vi "testFlushQueueTcpClient.vi"(8 "error in (no error)":errorcluster) -> (0 "error out":errorcluster)   [LabVIEW 2018]
doc: "Test the flushQueueTcpClient.vi."
uses:
  src/TcpServerBase/TcpServerBase.lvclass
  src/TcpServerBase/TcpServerBase.lvclass/TcpServerBase.ctl
  <vilib>/addons/_JKI Toolkits/Caraya/classes/Assert/Assert True.vi
  <vilib>/addons/_JKI Toolkits/Caraya/classes/Test/Test.lvclass
  <vilib>/addons/_JKI Toolkits/Caraya/classes/Assert/Assert.lvclass
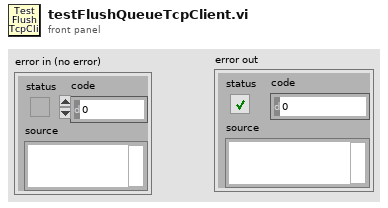
[diagram p1: front panel]
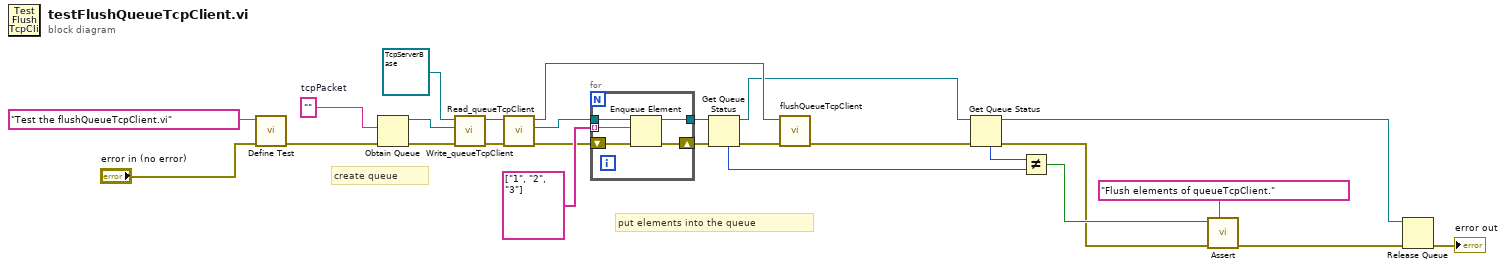
[diagram p0: block diagram]
diagram:
  w9 = ""  # tcpPacket
  # "put elements into the queue"
  # "create queue"
  n1 = call <vilib>:"Define Test.vi"("error in (no error)"="error in (no error)", "Label (VI Title)"="Test the flushQueueTcpClient.vi") -> ("error out"=w8:errorcluster)  [unwired: 9 in]
  n2 = Obtain Queue(element data type=w9, error in (no error)=w8) -> (queue out=w4:refnum<queue>, error out=w7:errorcluster)  [unwired: 3 in, 1 out]
  n3 = call "Write_queueTcpClient.vi"("error in (no error)"=w7, "queueTcpClient"=w4, "TcpServerBase in"=refnum<class "TcpServerBase.lvclass"> refnum ("TcpServerBase.lvclass")) -> ("error out"=w6:errorcluster, "TcpServerBase out"=w3:refnum<class "TcpServerBase.lvclass">)  [unwired: 7 in]
  n4 = call "Read_queueTcpClient.vi"("error in (no error)"=w6, "TcpServerBase in"=w3) -> ("error out"=w20:errorcluster, "queueTcpClient"=w19:refnum<queue>, "TcpServerBase out"=w18:refnum<class "TcpServerBase.lvclass">)  [unwired: 7 in]
  n5 = for {
    tunnel: string[] ["1", "2", "3"] -> [w30] mode=indexing
    tunnel: [w28] -> w17
    shift-right: [w29] -> w16
    shift-left: w20 -> [w31]
    tunnel: w19 -> [w27]
    n6 = Enqueue Element(queue=w27, element=w30, error in (no error)=w31) -> (queue out=w28:refnum<queue>, error out=w29:errorcluster)  [unwired: 1 in, 1 out]
  }
  n7 = Get Queue Status(queue=w17, error in (no error)=w16) -> (queue out=w13:refnum<queue>, error out=w15:errorcluster, # elements in queue=w11:i32)  [unwired: 1 in, 5 out]
  n8 = call "flushQueueTcpClient.vi"("error in (no error)"=w15, "TcpServerBase in"=w18) -> ("error out"=w14:errorcluster)  [unwired: 8 in, 1 out]
  n9 = Get Queue Status(queue=w13, error in (no error)=w14) -> (queue out=w2:refnum<queue>, error out=w1:errorcluster, # elements in queue=w12:i32)  [unwired: 1 in, 5 out]
  n10 = Not Equal?(x=w12, y=w11) -> (x != y?=w10:bool)
  n11 = call-poly <vilib>:"Assert.vi"("Label"="Flush elements of queueTcpClient.", "error in (no error)"=w1, "True?"=w10) -> ("error out"=w23:errorcluster)  [unwired: 8 in]
  n12 = Release Queue(queue=w2, error in (no error)=w23) -> (error out=→"error out":errorcluster)  [unwired: 1 in, 2 out]
